vi "SVL AC & DC Level (N Ch SGL Array).vi"(9 "window":u16(ring)=8 items=["None ", "Hanning", "Hamming", "Blackman-Harris", "Exact Blackman", "Blackman", "Flat Top", "4 Term B-Harris ", "7 Term B-Harris", "Low Sidelobe"], 11 "scaled signals [EU]":sgl[][](array[numeric])) -> (1 "DC levels [EU]":dbl[](array[numeric]) format="%0.2f", 2 "AC levels [EU rms]":dbl[](array[numeric]) format="%.8f", 3 "AC signals [EU]":sgl[][](array[numeric]))   [LabVIEW 2017]
doc: "Computes the AC level and DC level of a signal. Wire data to the <B>scaled signal [EU]</B> input to determine the polymorphic instance to use or manually select the instance."
uses:
  <vilib>/Analysis/baseanly.llb/Mean.vi
  <vilib>/Analysis/baseanly.llb/Mean (DBL).vi
  <vilib>/Analysis/baseanly.llb/Std Deviation and Variance.vi
  <vilib>/Analysis/0measdsp.llb/Scaled Time Domain Window.vi
  <vilib>/Analysis/0measdsp.llb/Scaled Time Domain Window (DBL).vi
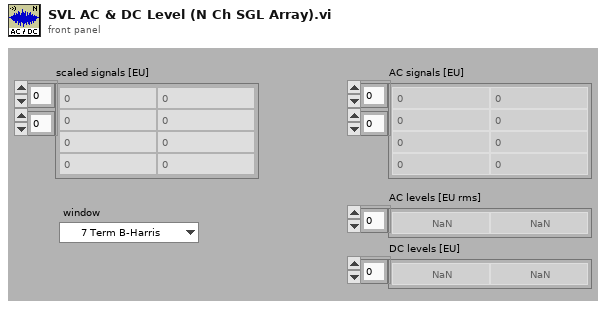
[diagram p1: front panel]
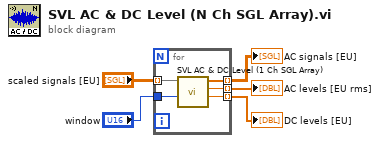
[diagram p0: block diagram]
diagram:
  n1 = for {
    tunnel: "scaled signals [EU]" -> [w10] mode=indexing
    tunnel: [w9] -> w4 mode=indexing
    tunnel: [w8] -> w3 mode=indexing
    tunnel: [w7] -> w2 mode=indexing
    tunnel: "window" -> [w6]
    n2 = call <vilib>:"SVL AC & DC Level (1 Ch SGL Array).vi"("window"=w6, "scaled signal [EU]"=w10) -> ("DC level [EU]"=w7:dbl, "AC level [EU rms]"=w8:dbl, "AC signal [EU]"=w9:sgl[])  [unwired: 7 in]
  }
  "AC levels [EU rms]" <- w3
  "AC signals [EU]" <- w4
  "DC levels [EU]" <- w2
